vi "ConfirmElementRequestDecode.vi"(1 "Payload":string) -> (0 "RequestId":u8)   [LabVIEW 2009]
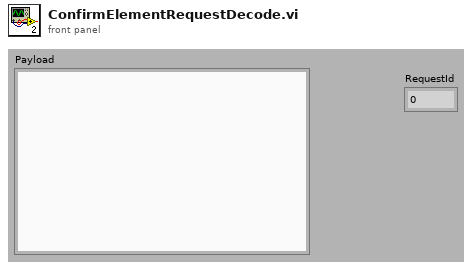
[diagram p1: front panel]
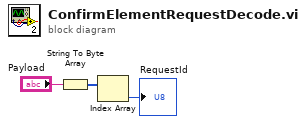
[diagram p0: block diagram]
diagram:
  n1 = String To Byte Array(string="Payload") -> (unsigned byte array=w2:u8[])
  n2 = Index Array(array=w2) -> (element=→"RequestId":u8)  [unwired: 1 in]
